vi "find_type.vi"(10 "type_string":string, 11 "error in (no error)":errorcluster) -> (2 "type_enum":T1=enum."application_pc", 3 "error out":errorcluster)   [LabVIEW 2015, in "lv-build.lvlib"]
uses:
  lv-build.lvlib
  public/_controls/build_type.ctl
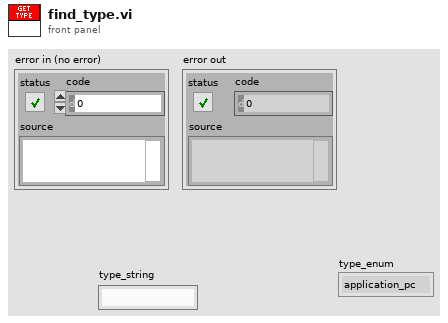
[diagram p1: front panel]
types:
  T1 = typedef "lv-build.lvlib/build_type.ctl" = enum16{"<build_type>", "application_pc", "application_rt", "installer", "llb", "lvlibp", "zip", "fpga", "<null>"}
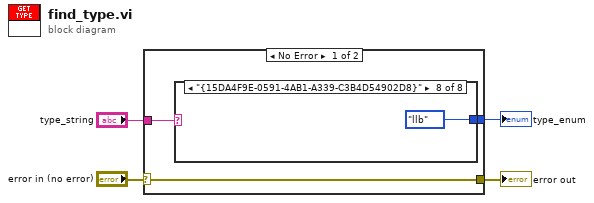
[diagram p0: block diagram]
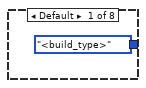
[diagram p2: hidden frame]
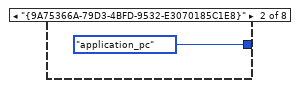
[diagram p3: hidden frame]
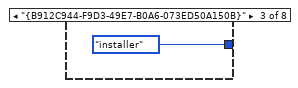
[diagram p4: hidden frame]
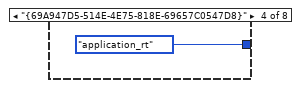
[diagram p5: hidden frame]
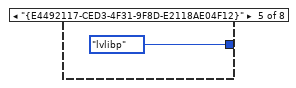
[diagram p6: hidden frame]
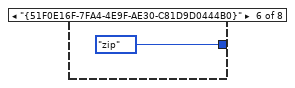
[diagram p7: hidden frame]
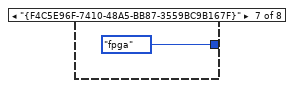
[diagram p8: hidden frame]
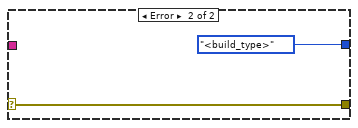
[diagram p9: hidden frame]
diagram:
  n1 = case shown="No Error" "error in (no error)" {
    selector: "error in (no error)" -> [w5 w17]
    tunnel: "type_string" -> [w7 _]
    tunnel: [w6 build_type."<build_type>" ("Type out")] -> w3
    tunnel: [w5 w17] -> w1
    frame No Error {
      n2 = case shown="\"{15DA4F9E-0591-4AB1-A339-C3B4D54902D8}\"" w7 {
        tunnel: [build_type."<build_type>" ("Type out") build_type."application_pc" ("Type out") build_type."installer" ("Type out") build_type."application_rt" ("Type out") build_type."lvlibp" ("Type out") build_type."zip" ("Type out") build_type."fpga" ("Type out") build_type."llb" ("Type out")] -> w6
        frame Default {
        }
        frame "{9A75366A-79D3-4BFD-9532-E3070185C1E8}" {
        }
        frame "{B912C944-F9D3-49E7-B0A6-073ED50A150B}" {
        }
        frame "{69A947D5-514E-4E75-818E-69657C0547D8}" {
        }
        frame "{E4492117-CED3-4F31-9F8D-E2118AE04F12}" {
        }
        frame "{51F0E16F-7FA4-4E9F-AE30-C81D9D0444B0}" {
        }
        frame "{F4C5E96F-7410-48A5-BB87-3559BC9B167F}" {
        }
        frame "{15DA4F9E-0591-4AB1-A339-C3B4D54902D8}" {
        }
      }
    }
    frame Error {
    }
  }
  "error out" <- w1
  "type_enum" <- w3
